vi "DataMap.vi"(2 "Value In":string, 3 "Name":string, 4 "Data In":string[][](table)) -> (0 "Value Out":string, 1 "Data Out":string[][](table))   [LabVIEW 2011]
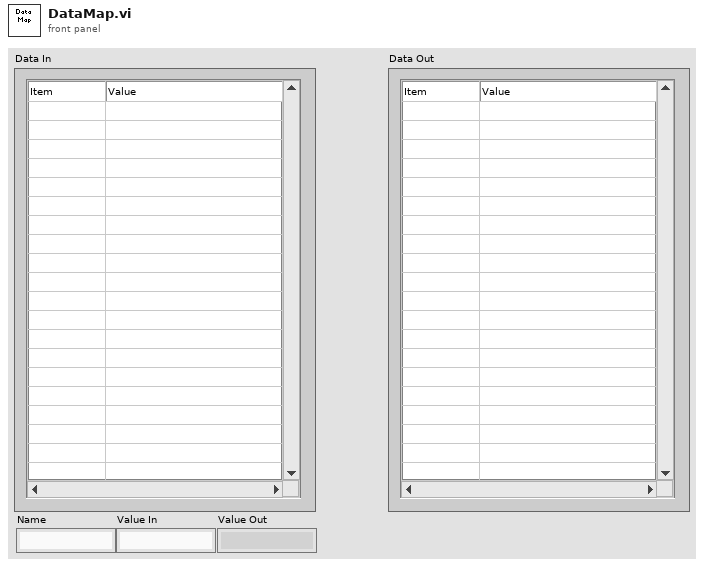
[diagram p1: front panel]
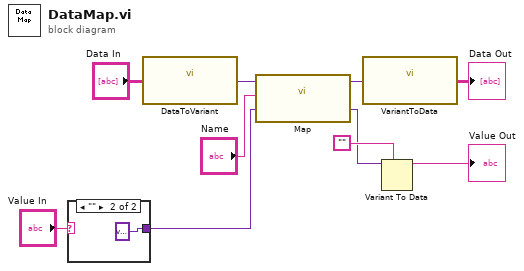
[diagram p0: block diagram]
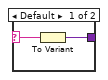
[diagram p2: hidden frame]
diagram:
  n1 = case shown="\"\"" "Value In" {
    selector: "Value In" -> [w12 _]
    tunnel: [w11 variant ("variant")] -> w6
    frame Default {
      n2 = To Variant(anything=w12) -> (Variant=w11:variant)
    }
    frame "" {
    }
  }
  n3 = call "DataToVariant.vi"("Data"="Data In") -> ("Variant"=w5:variant)
  n4 = call "Map.vi"("Value In"=w6, "Name"="Name", "Map In"=w5) -> ("Value Out"=w2:variant, "Map Out"=w4:variant)
  n5 = call "VariantToData.vi"("Variant"=w4) -> ("Data"=→"Data Out":string[][])
  n6 = Variant To Data(type="", Variant=w2) -> (data=→"Value Out":string)  [unwired: 1 in, 1 out]
